vi "Bundle.vi"(8 "error in (no error)":errorcluster, 9 "Hander Index":i32, 10 "Aquirer Lock":T1, 11 "Multi Instrument Handler in":refnum<class "Multi Instrument Handler.lvclass">) -> (0 "error out":errorcluster, 3 "Multi Instrument Handler out":refnum<class "Multi Instrument Handler.lvclass">)   [LabVIEW 2020, in "Instrument Handler.lvlib" / "Multi Instrument Handler.lvclass"]
doc: "Write the Aquirer Lock semaphore and the Handler Index to the Multi Instrument Handler."
uses:
  Multi Instrument Handler.lvclass
  Multi Instrument Handler.lvclass/Multi Instrument Handler.ctl
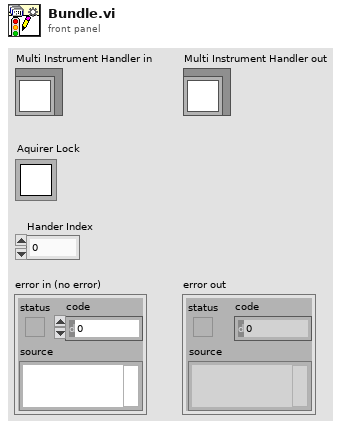
[diagram p1: front panel]
types:
  T1 = typedef "Semaphore RefNum" = refnum<k1>
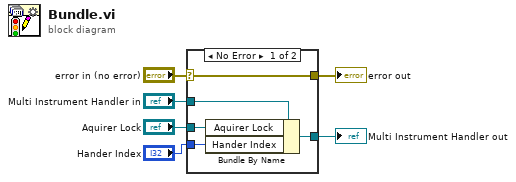
[diagram p0: block diagram]
diagram:
  n1 = case shown="No Error" "error in (no error)" {
    selector: "error in (no error)" -> [w11 w12]
    tunnel: [w11 w12] -> w5
    tunnel: [w9 w13] -> w3
    tunnel: "Multi Instrument Handler in" -> [w10 w13]
    tunnel: "Aquirer Lock" -> [w8 _]
    tunnel: "Hander Index" -> [w7 _]
    frame No Error {
      n2 = Bundle By Name(cluster=w10, "Aquirer Lock"=w8, "Hander Index"=w7) -> (w9:refnum<class "Multi Instrument Handler.lvclass">)
    }
    frame Error {
    }
  }
  "error out" <- w5
  "Multi Instrument Handler out" <- w3
